vi "Write 1Chan 1Sample SGL.vi"(8 "error in (no error)":errorcluster, 10 "data":dbl, 11 "Analog Output in":refnum<class "Analog output.lvclass">) -> (0 "error out":errorcluster, 3 "Analog Output out":refnum<class "Analog output.lvclass">)   [LabVIEW 2009, in "MicroDAQ.lvlib" / "Analog output.lvclass"]
doc: "Writes const value to one channel."
uses:
  <instrlib>/MicroDAQ/Channel/Analog Output/Analog output.lvclass
  <instrlib>/MicroDAQ/Channel/Analog Output/Analog output.lvclass/Analog output.ctl
  <instrlib>/MicroDAQ/Channel/Channel.lvclass
  <instrlib>/MicroDAQ/Mlink library wraper/mlink.lvlib
  <instrlib>/MicroDAQ/MicroDAQ.lvlib
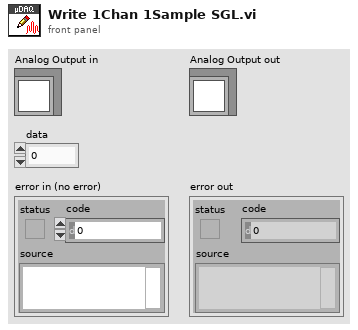
[diagram p1: front panel]
types:
  T1 = typedef "MicroDAQ.lvlib/Analo Range Enum.ctl" = enum16{"±10V", "0-10V", "±5V", "0-5V", "±5.12V", "±2.56V", "±2.5V", "±2V", "±1.24V", "±0.64V"}
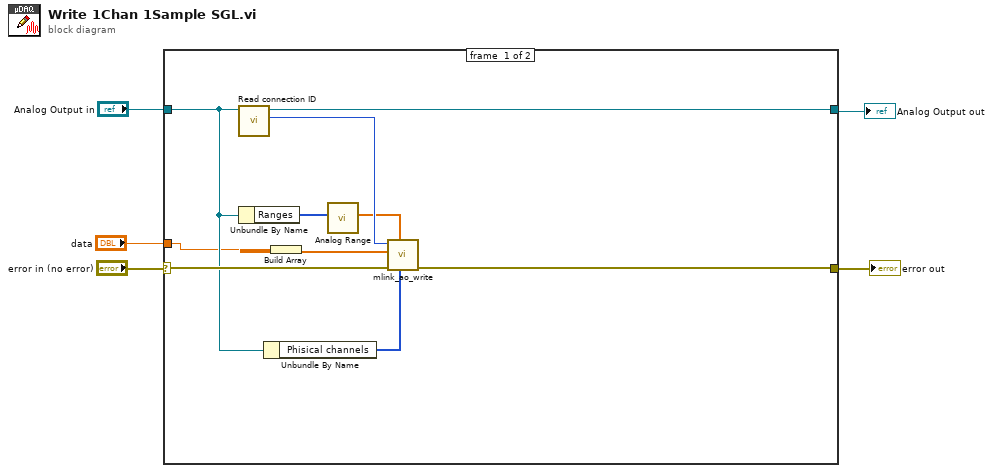
[diagram p0: block diagram]
diagram:
  n1 = case shown="No Error" "error in (no error)" {
    selector: "error in (no error)" -> [w13 w17]
    tunnel: [w7 w17] -> w4
    tunnel: [w15 w16] -> w2
    tunnel: "Analog Output in" -> [w12 w16]
    tunnel: "data" -> [w10 _]
    frame #0 {
      n2 = call <instrlib>:"Read connection ID.vi"("Task in"=w12) -> ("connection ID"=w14:i32, "Task out"=w15:refnum<class "Analog output.lvclass">)  [unwired: 9 in]
      n3 = Unbundle By Name(w12) -> ("Ranges"=w9:T1[])
      n4 = Unbundle By Name(w12) -> ("Phisical channels"=w8:u8[])
      n5 = Build Array(w10) -> (w11:dbl[])
      n6 = call <instrlib>:"Analog Range.vi"("ranges in"=w9) -> ("range Array out"=w6:dbl[])  [unwired: 10 in]
      n7 = call <instrlib>:"mlink_ao_write.vi"("channels"=w8, "range"=w6, "error in (no error)"=w13, "data"=w11, "connection ID"=w14) -> ("error out"=w7:errorcluster)  [unwired: 5 in, 1 out]
    }
    frame #1 {
    }
  }
  "error out" <- w4
  "Analog Output out" <- w2
